vi "WgHOut2Dummy.vi"(2 "error in (no error)":errorcluster) -> (0 "error out":errorcluster)   [LabVIEW 2009]
doc: "Waveguide switch - H Out - connect to Dummy"
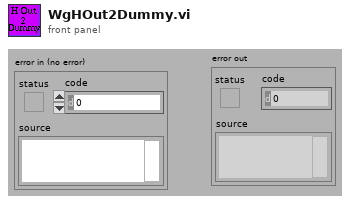
[diagram p1: front panel]
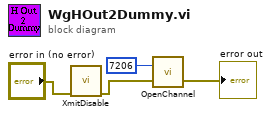
[diagram p0: block diagram]
diagram:
  n1 = call "XmitDisable.vi"("error in (no error)"="error in (no error)") -> ("error out"=w1:errorcluster)  [unwired: 1 in, 5 out]
  n2 = call "OpenChannel.vi"("error in (no error)"=w1, "Channel ID"=7206) -> ("error out"=→"error out":errorcluster)  [unwired: 1 in]
